vi "Dispense X Gallons.vi"() -> ()   [LabVIEW 2009]
uses:
  ChannelSettings.ctl
  Intellifaucet/Intellfaucet Mode.ctl
panel:
  out "PreviousRate 2":dbl
  in  "Gallons to Dispense 2":dbl
  out "Waveform Chart":dbl(graph)
  in  "Temperature(F)":dbl=58.0
  in  "Percent Flow":dbl=30.0
  out "Elapsed Time(s)2":dbl
  out "Gallons 2":dbl
  in  "Gallons to Dispense":dbl
  in  "Stop":bool
  out "Gallons":dbl
  out "Elapsed Time(s)":dbl
  out "PreviousRate":dbl
  out "Current Rate":dbl
  out "Error Out":errorcluster
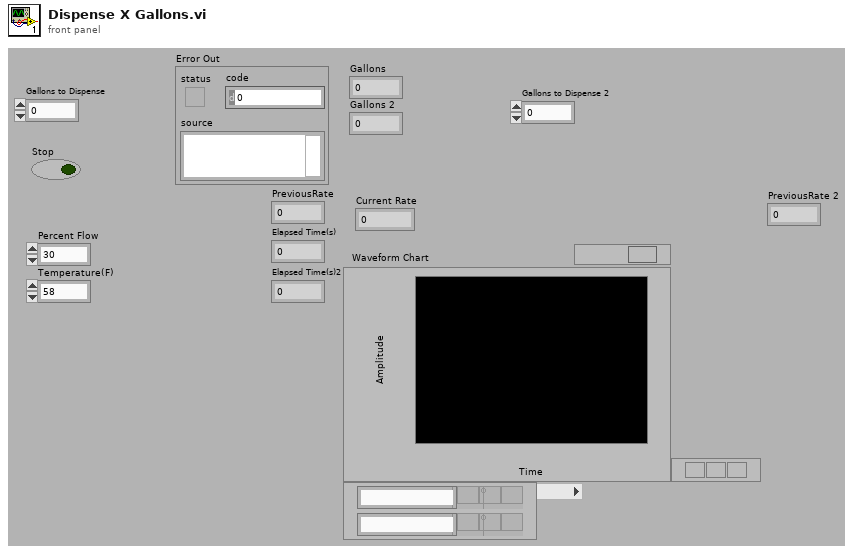
[diagram p1: front panel]
types:
  T1 = typedef "Intellfaucet Mode.ctl" = enum16{"Adjust Temp", "Adjust Flow", "Start Flow", "Stop Flow"}
  T2 = typedef "Semaphore RefNum" = refnum<k1>
  T3 = typedef "ChannelSettings.ctl" = u16
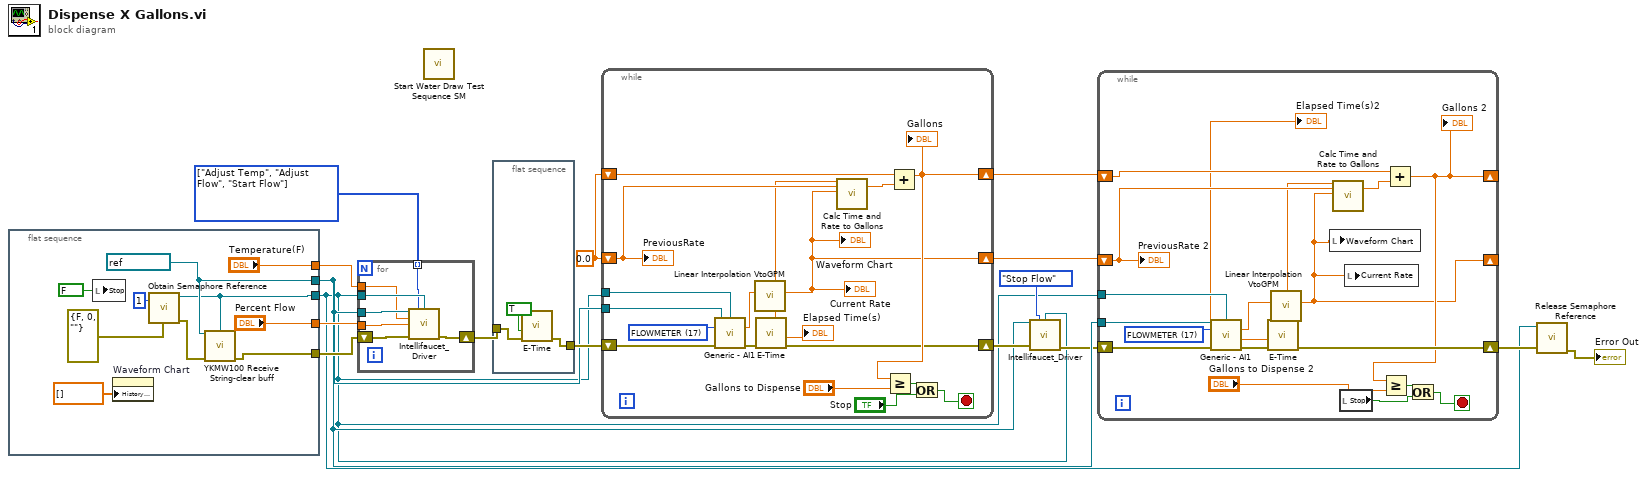
[diagram p0: block diagram]
diagram:
  w12 = T1[] [enum."Adjust Temp", enum."Adjust Flow", enum."Start Flow"] items=["Adjust Temp", "Adjust Flow", "Start Flow", "Stop Flow"]
  w15 = 0.0 ("Value")
  n1 = flat-sequence {
    tunnel: [w18] -> w1
    tunnel: [w19] -> w4
    tunnel: ["Percent Flow"] -> w11
    tunnel: ["Temperature(F)"] -> w10
    tunnel: [w20] -> w9
    frame #0 {
      w19 = refnum<visa-resource-name> "MW100" ("VISA session")
      n2 = local write "Stop"(FALSE ("Stop")) -> ()
      n3 = property on="Waveform Chart" class="WFChart (strict)"("History Data"=dbl[] []) -> ()  [unwired: 2 in, 2 out]
      n4 = call <vilib>:"Obtain Semaphore Reference.vi"("error in (no error)"=errorcluster {"status"=FALSE, "code"=0, "source"=""}, "size (1)"=1) -> ("error out"=w21:errorcluster, "semaphore"=w18:T2)  [unwired: 3 in, 1 out]
      n5 = call "YKMW100 Receive String-clear buff.vi"("VISA session"=w19, "Semiphore"=w18, "error in (no error)"=w21) -> ("error out"=w20:errorcluster)  [unwired: 10 in, 2 out]
    }
  }
  n6 = for {
    tunnel: w1 -> [w31]
    tunnel: w4 -> [w30]
    tunnel: w12 -> [w29] mode=indexing
    tunnel: w11 -> [w28]
    tunnel: w10 -> [w27]
    shift-right: [w32] -> w14
    shift-left: w9 -> [w33]
    n7 = call "Intellifaucet_Driver.vi"("VISA session"=w30, "Mode"=w29, "Semiphore"=w31, "Temperature(F)"=w27, "Percent Flow"=w28, "Error In"=w33) -> ("Error Out"=w32:errorcluster)  [unwired: 8 in, 1 out]
  }
  n8 = call "Start Water Draw Test Sequence SM.vi"() -> ()  [unwired: 12 in, 4 out]
  n9 = flat-sequence {
    tunnel: w14 -> [w34]
    tunnel: [w35] -> w8
    frame #0 {
      n10 = call "E-Time.vi"("error in (no error)"=w34, "Reset"=TRUE) -> ("error out"=w35:errorcluster)  [unwired: 7 in, 2 out]
    }
  }
  n11 = while {
    tunnel: w4 -> [w53]
    shift-right: [w39] -> w13
    shift-left: w8 -> [w52]
    tunnel: w1 -> [w51]
    shift-right: [w41] -> w5
    shift-left: w15 -> [w43]
    shift-right: [w45] -> w6
    shift-left: w15 -> [w50]
    stop <- w47 stop-if-true
    w54 = T3 17 items=["RTD_IN", "RTD_OUT", "RTD_AMB", "Tc_1", "Tc_2", "Tc_3", "Tc_4", "Tc_5", "Tc_6", "Tc_down", "Pres_HI1", "Pres_HI2", "Pres_LOW", "VLV_IN", "VLV_DUMP", "VLV_OUT", "PWR_MAIN", "FLOWMETER", "4-20_OUT", "HEATER_TOP", "HEATER_BOT", "COMPRESSOR", "DRM_LOW", "DRM_HIGH", "INTF_TEMPFLO", "INTF_READY", "INTF_START", "INTF_STOP"] ("Channel_Enum")
    n12 = call "Generic - AI1.vi"("MW100"=w53, "Semiphore"=w51, "Channel_Enum"=w54, "Error In"=w52) -> ("Value"=w44:dbl, "Error Out"=w40:errorcluster)  [unwired: 9 in, 1 out]
    n13 = call "Linear Interpolation VtoGPM.vi"("V"=w44) -> ("GPM"=w41:dbl)  [unwired: 10 in]
    "Current Rate" <- w41
    "Waveform Chart" <- w41
    n14 = call "E-Time.vi"("error in (no error)"=w40) -> ("error out"=w39:errorcluster, "Elapsed Time (sec)"=→"Elapsed Time(s)":dbl, "Time Since Last Run (sec)"=w38:dbl)  [unwired: 8 in]
    n15 = call "Calc Time and Rate to Gallons.vi"("Elapsed Time(s)"=w38, "Previous Rate"=w43, "Current Rate"=w41) -> ("Gallons"=w42:dbl)  [unwired: 16 in]
    n16 = Add(x=w50, y=w42) -> (x+y=w45:dbl)
    "Gallons" <- w45
    n17 = Greater Or Equal?(x=w45, y="Gallons to Dispense") -> (x >= y?=w49:bool)
    n18 = Or(x=w49, y="Stop") -> (x .or. y?=w47:bool)
    "PreviousRate" <- w43
  }
  n19 = call "Intellifaucet_Driver.vi"("VISA session"=w4, "Mode"=Intellfaucet_Mode."Stop Flow", "Semiphore"=w1, "Error In"=w13) -> ("Error Out"=w3:errorcluster)  [unwired: 10 in, 1 out]
  n20 = while {
    tunnel: w4 -> [w71]
    shift-right: [w60] -> w2
    shift-left: w3 -> [w70]
    tunnel: w1 -> [w69]
    shift-right: [w55] -> _
    shift-left: w5 -> [w63]
    shift-right: [w57] -> _
    shift-left: w6 -> [w68]
    stop <- w66 stop-if-true
    w72 = T3 17 items=["RTD_IN", "RTD_OUT", "RTD_AMB", "Tc_1", "Tc_2", "Tc_3", "Tc_4", "Tc_5", "Tc_6", "Tc_down", "Pres_HI1", "Pres_HI2", "Pres_LOW", "VLV_IN", "VLV_DUMP", "VLV_OUT", "PWR_MAIN", "FLOWMETER", "4-20_OUT", "HEATER_TOP", "HEATER_BOT", "COMPRESSOR", "DRM_LOW", "DRM_HIGH", "INTF_TEMPFLO", "INTF_READY", "INTF_START", "INTF_STOP"] ("Channel_Enum")
    n21 = call "Generic - AI1.vi"("MW100"=w71, "Semiphore"=w69, "Channel_Enum"=w72, "Error In"=w70) -> ("Value"=w64:dbl, "Error Out"=w61:errorcluster)  [unwired: 9 in, 1 out]
    n22 = call "E-Time.vi"("error in (no error)"=w61) -> ("error out"=w60:errorcluster, "Elapsed Time (sec)"=→"Elapsed Time(s)2":dbl, "Time Since Last Run (sec)"=w59:dbl)  [unwired: 8 in]
    n23 = call "Linear Interpolation VtoGPM.vi"("V"=w64) -> ("GPM"=w55:dbl)  [unwired: 10 in]
    n24 = local write "Waveform Chart"(w55) -> ()
    n25 = call "Calc Time and Rate to Gallons.vi"("Elapsed Time(s)"=w59, "Previous Rate"=w63, "Current Rate"=w55) -> ("Gallons"=w62:dbl)  [unwired: 16 in]
    n26 = local read "Stop"() -> (w56:bool)
    n27 = local write "Current Rate"(w55) -> ()
    n28 = Add(x=w68, y=w62) -> (x+y=w57:dbl)
    "Gallons 2" <- w57
    n29 = Greater Or Equal?(x=w57, y="Gallons to Dispense 2") -> (x >= y?=w67:bool)
    n30 = Or(x=w67, y=w56) -> (x .or. y?=w66:bool)
    "PreviousRate 2" <- w63
  }
  n31 = call <vilib>:"Release Semaphore Reference.vi"("error in (no error)"=w2, "semaphore"=w1) -> ("error out"=→"Error Out":errorcluster)  [unwired: 8 in, 1 out]
